vi "load_controller_a.vi"(0 "Load 1":bool, 1 "Load 2":bool, 2 "Load 3":bool, 3 "Load 4":bool, 4 "First Visible Index":u32) -> ()   [LabVIEW 2017]
panel:
  out "Load":bool
  out "Index":dbl
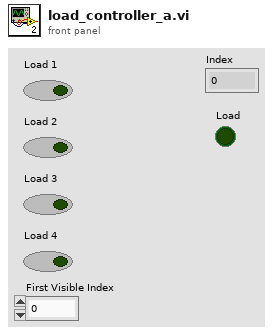
[diagram p1: front panel]
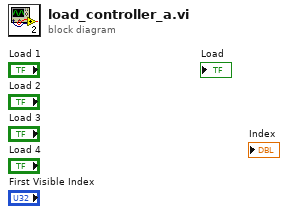
[diagram p0: block diagram]
diagram:
